vi "main_interface-while-2635_8.3_ZS.vi"() -> ()   [LabVIEW 2014]
uses:
  Instance           1 34Saved   main_interface-while-2635. .vi
  Instance           2 34Saved   main_interface-while-2635. .vi
  Instance           3 34Saved   main_interface-while-2635. .vi
panel:
  out "Vmax":dbl
  out "Jmax":dbl
  in  "Collate Files":bool
  in  "Finger Number":dbl=1.0 min=1.0 max=5.0 step=1.0
  in  "Solar Cell Number":dbl=1.0 min=1.0 max=12.0 step=1.0 format="%0#2_2g"
  in  "Dark Current?":bool
  out "size(s)":i32
  in  "Speed":dbl=1.0
  in  "Serial Configuration":T1={"Baud Rate"=115200, "Parity"=0, "Data Bits"=8, "Stop Bits"=10, "Flow Control"=0} {"Flow Control" items=["None", "XON/XOFF", "RTS/CTS", "XON/XOFF & RTS/CTS", "DTR/DSR", "XON/XOFF & DTR/DSR"]; "Stop Bits" items=["1.0"=10, "1.5"=15, "2.0"=20]; "Data Bits" items=["7"=7, "8"=8]; "Parity" items=["None", "Odd", "Even", "Mark", "Space"]; "Baud Rate" items=["300"=300, "600"=600, "1200"=1200, "2400"=2400, "4800"=4800, "9600"=9600, "19200"=19200]}
  in  "Tab Control":enum32{"Linear Scale", "Log scale"}(tab)
  out "XY Graph":cluster{dbl[], dbl[]}(graph)
  out "XY Graph 2":cluster{dbl[], dbl[]}(graph)
  in  "Start Measurement?":bool
  out "Read Data!":string
  in  "Read File?":bool
  out "S_J_Output (mA/cm^2)":string
  out "J":dbl[](array[numeric])
  out "current_density":dbl[](array[numeric])
  in  "The compliance current (A)":dbl=0.5
  out "stop":bool
  in  "Cancel Measurement?":bool
  out "voltage":dbl[](array[numeric])
  out "current":dbl[](array[numeric])
  out "|voltage|":dbl[](array[numeric])
  out "power":dbl[](array[numeric])
  out "|current|":dbl[](array[numeric])
  out "Measurement Completed?":bool
  in  "Completed, Exit?":bool
  in  "Save to Text file?":bool
  out "path":path
  out "finish":bool
  out "Pmax":dbl
  out "FF":dbl
  out "Isc":dbl
  out "Voc":dbl
  in  "Device Area (cm^2)":dbl=0.06 caption="Step Size (V)" format="%#_6f"
  out "Jsc":dbl
  out "PCE":dbl
  in  "Light  Intensity (mW/cm^2)":dbl=100.0 caption="Step Size (V)" min=2.0
  out "Nth. of Step":i32
  out "error out":errorcluster
  out "S_V_Output (V)":string
  out "S_I_Output (A)":string
  in  "VISA resource name":refnum<visa-resource-name>="COM1"
  out "Voltage increment":dbl
  in  "Final Voltage":dbl=1.0 caption="Final Voltage (V)"
  in  "Step Number":i32=150 caption="Step Size (V)" min=2
  in  "Initial Voltage":dbl=-0.5 caption="Initial Voltage (V)"
  # "(The result will be \nmore accuracy if the\nstep number is larger),"
  # "(0.01-10,the smallar\nvalue,the faster speed)"
  # "Data has been saved!"
  # "To automatically create an Excel Report. \nClick Collate Files and choose all the text files \nwhoose data you want to include in the report"
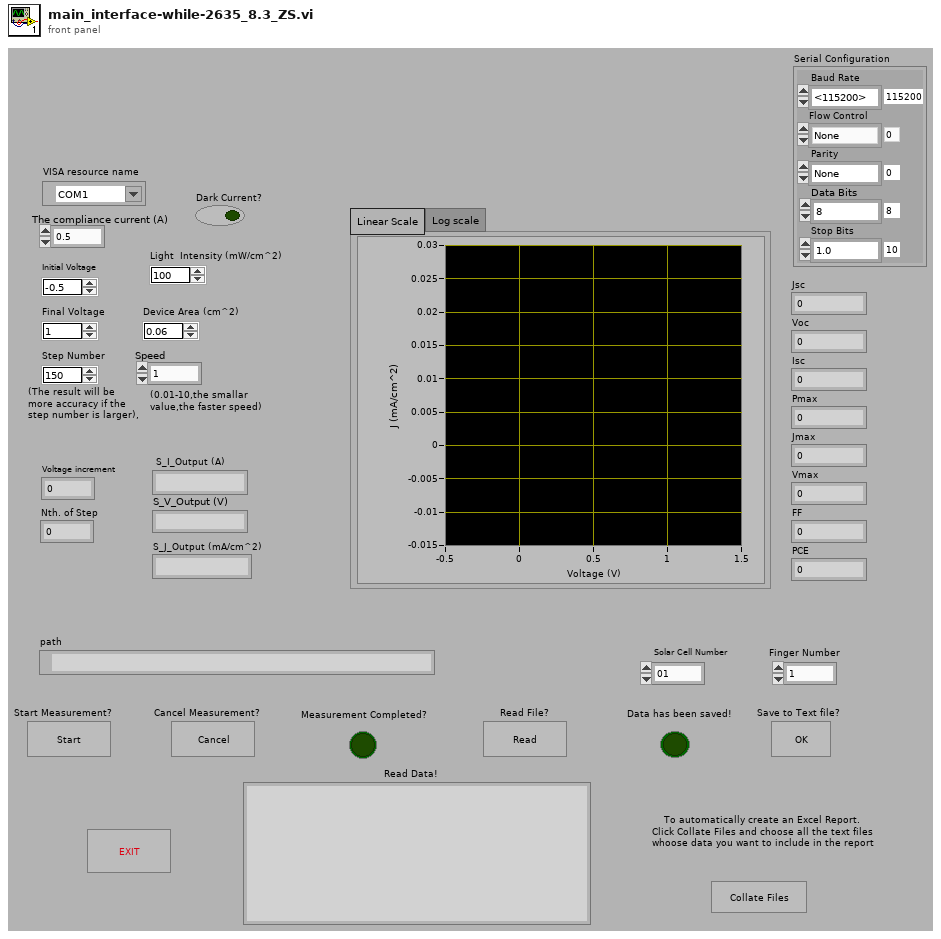
[diagram p1: front panel]
types:
  T1 = cluster{"Baud Rate":u32, "Parity":u16, "Data Bits":u16, "Stop Bits":u16, "Flow Control":u16}
  T2 = enum16{"open", "replace", "create", "open or create", "replace or create", "replace or create with confirmation"}
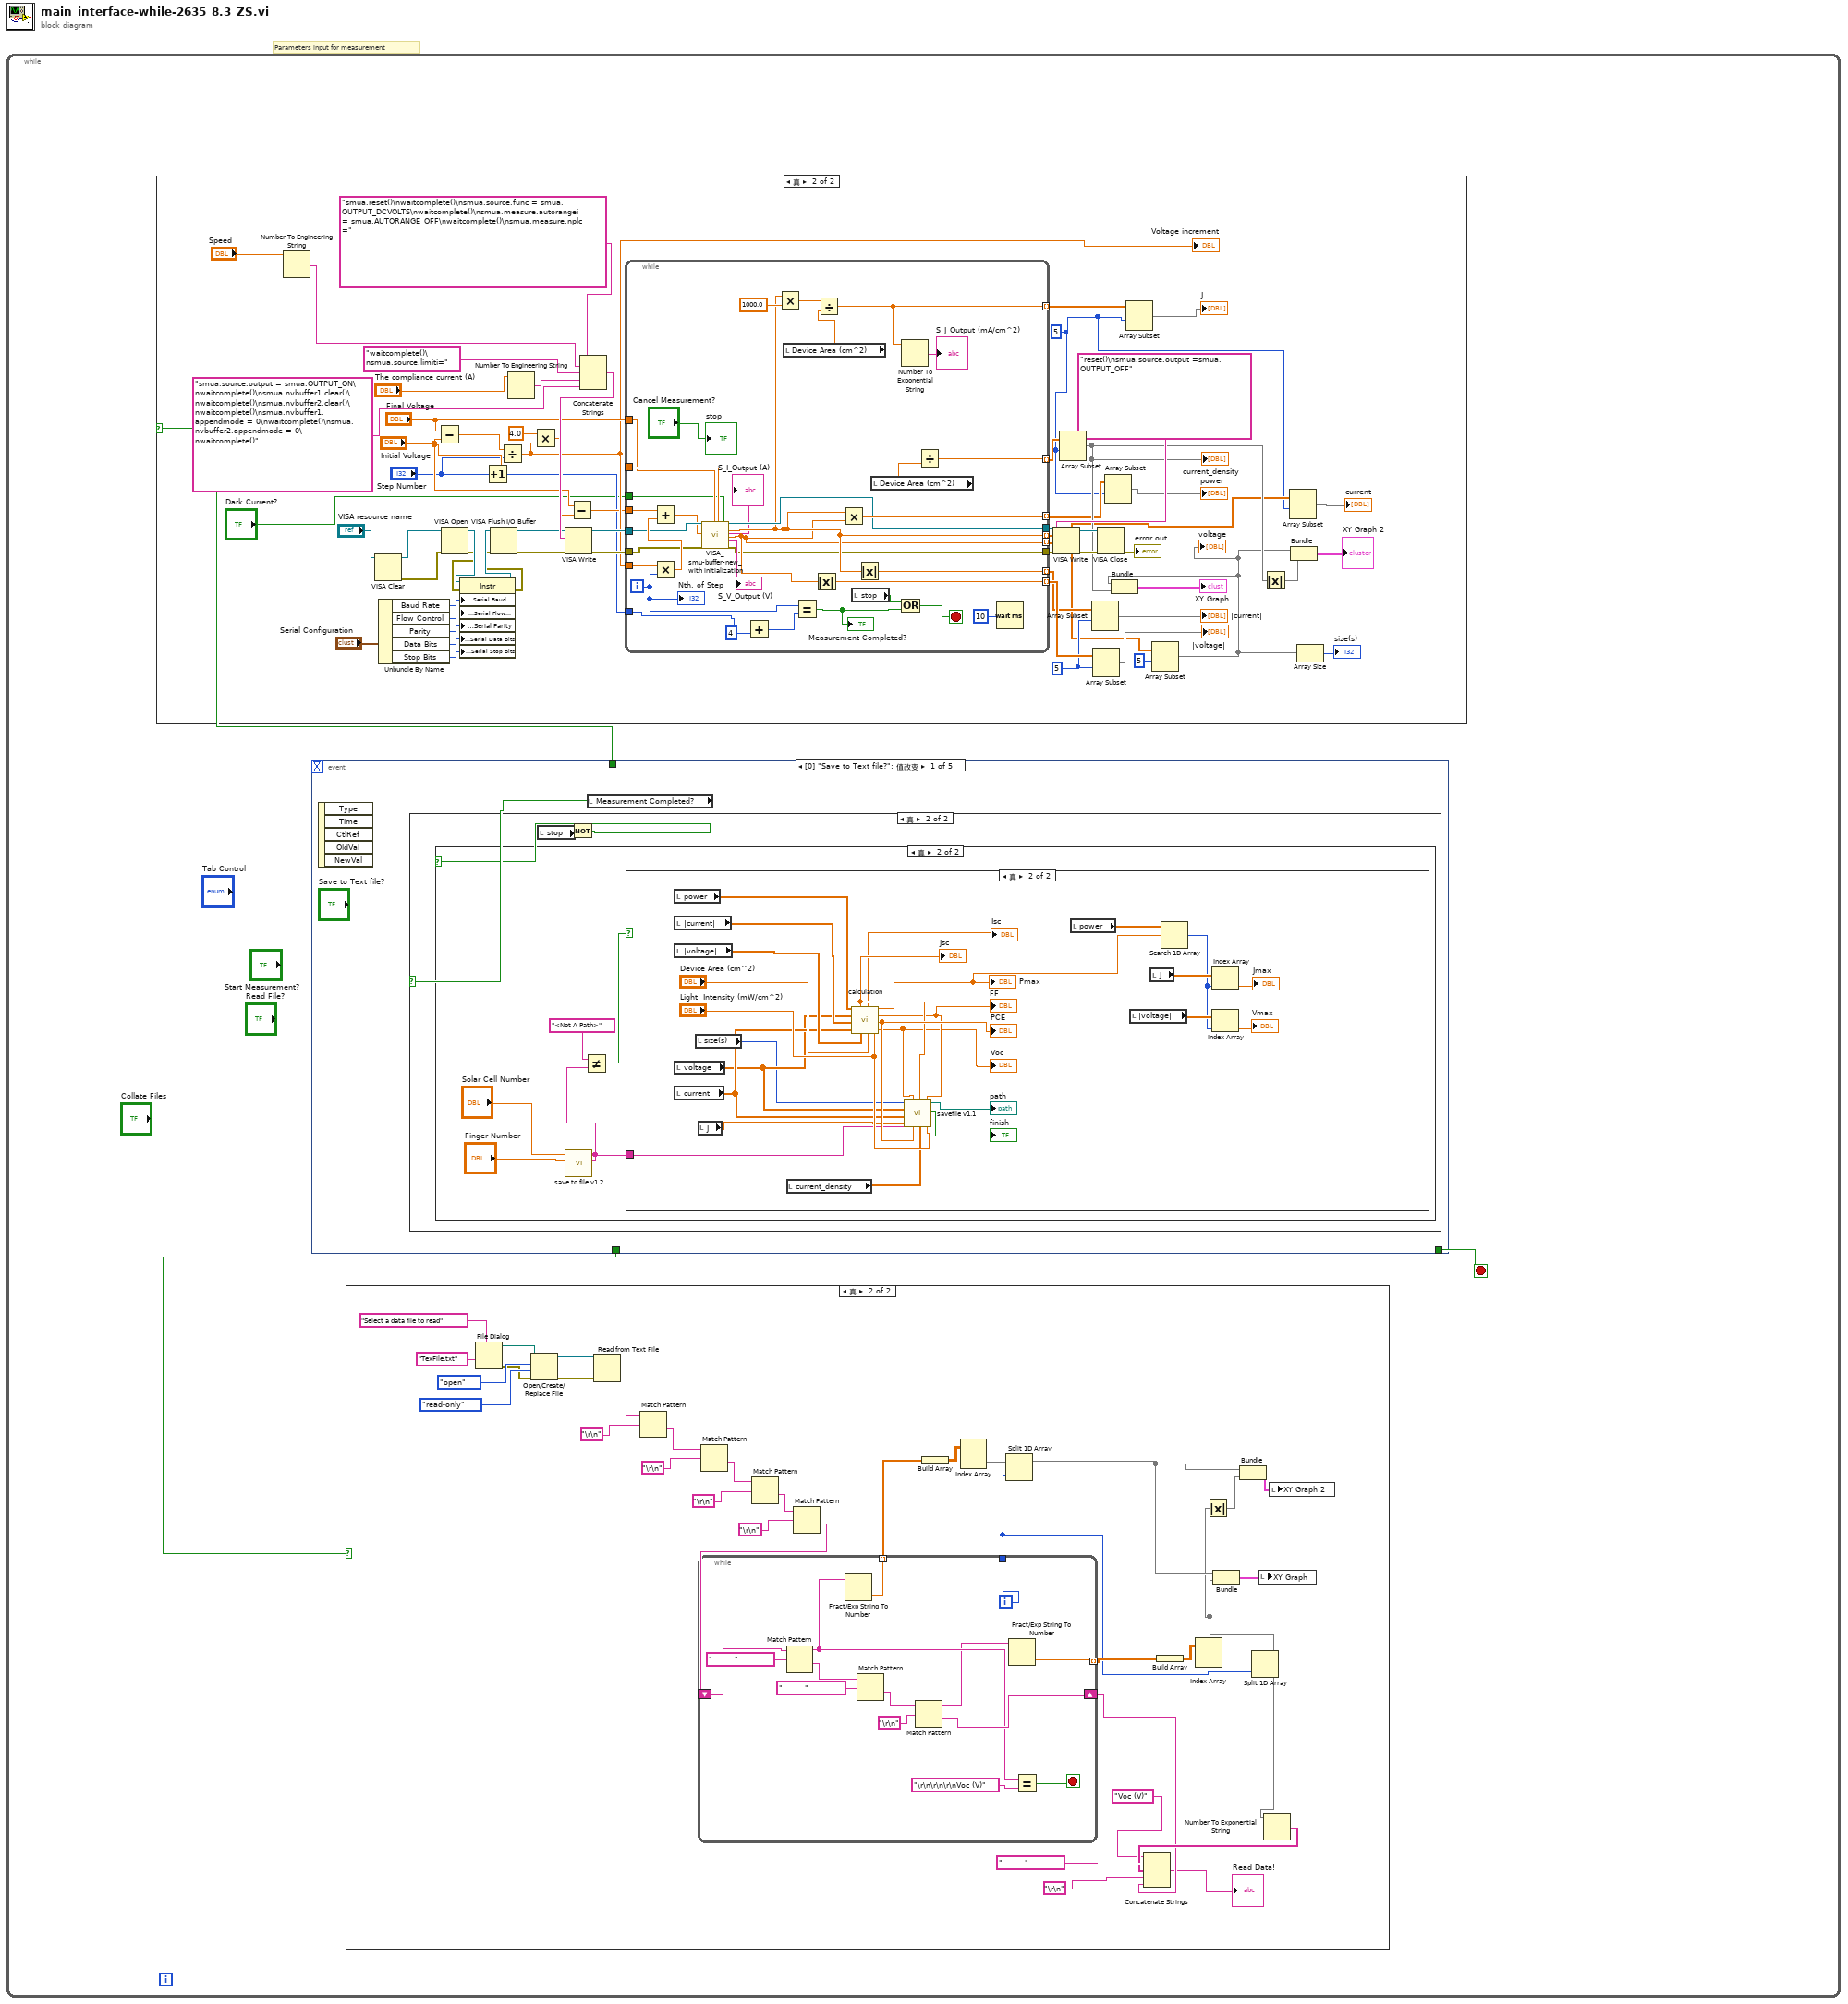
[diagram p0: block diagram]
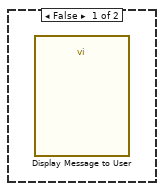
[diagram p4: hidden frame]
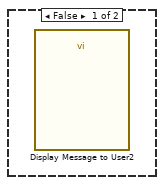
[diagram p5: hidden frame]
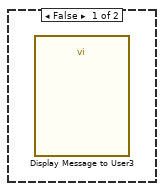
[diagram p6: hidden frame]
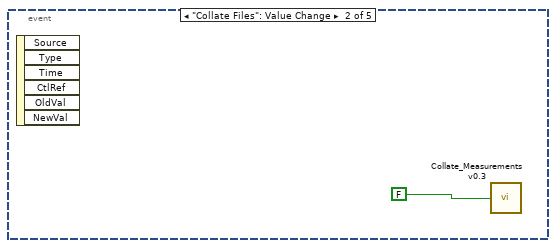
[diagram p7: hidden frame]
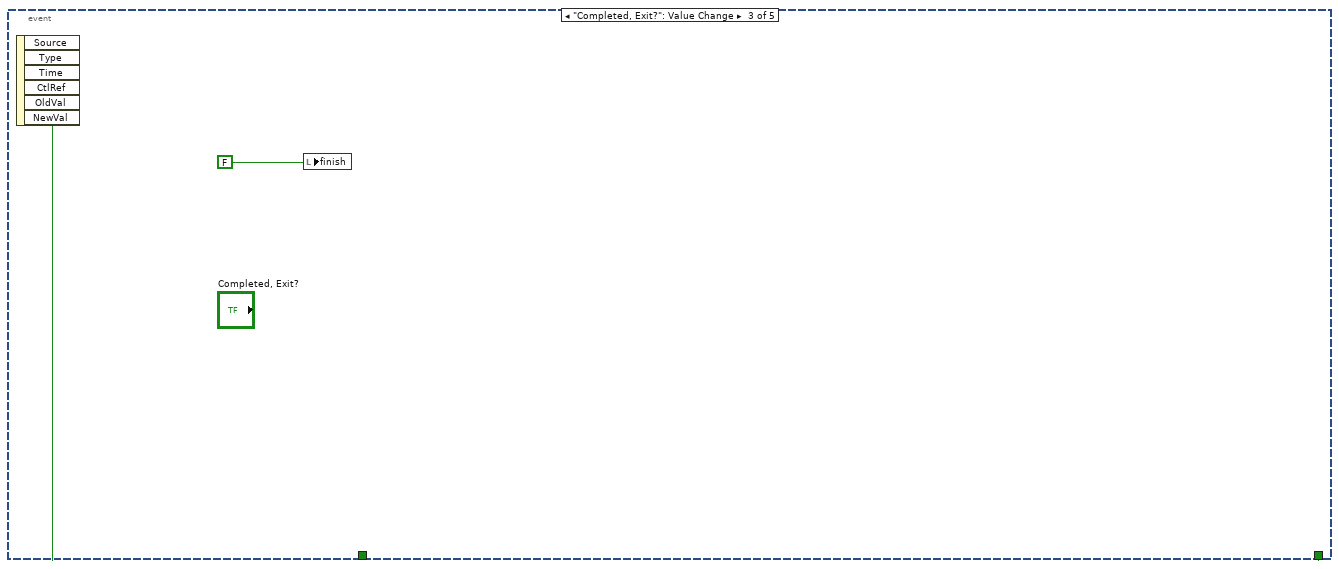
[diagram p8: hidden frame]
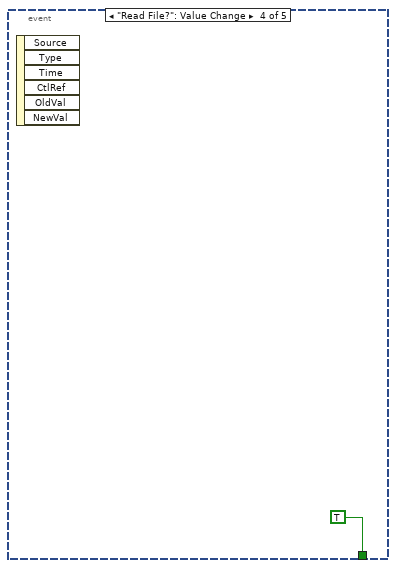
[diagram p9: hidden frame]
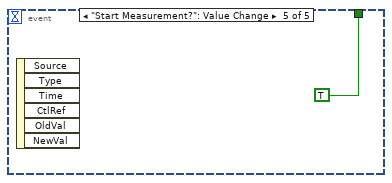
[diagram p10: hidden frame]
diagram:
  # "Parameters input for measurement"
  n1 = while {
    stop <- w3 stop-if-true
    n2 = event shown="[0] \"Save to Text file?\": 值改变" {
      selector: _ -> [_ _ _ _ _]
      dyn-events: _ -> [_ _ _ _ _]
      timeout: _ -> [_ _ _ _ _]
      tunnel: [_ _ w185 _ _] -> w3
      tunnel: [_ _ _ TRUE _] -> w2
      tunnel: [_ _ _ _ TRUE] -> w1
      event "Save to Text file?": Value Change {
        n3 = event-data() -> ()  [unwired: 6 out]
        n4 = local read "Measurement Completed?"() -> (w150:bool)
        n5 = case shown="真" w150 {
          frame False {
            n6 = call "Display Message to User"() -> ()  [unwired: 3 in, 9 out]
          }
          frame True {
            n7 = local read "stop"() -> (w152:bool)
            n8 = Not(x=w152) -> (.not. x?=w151:bool)
            n9 = case shown="真" w151 {
              frame False {
                n10 = call "Display Message to User2"() -> ()  [unwired: 3 in, 9 out]
              }
              frame True {
                n11 = call "save to file v1.2.vi"("Trial Number"="Finger Number", "Solar Cell Number"="Solar Cell Number") -> ("Path"=w155:string)  [unwired: 9 out]
                n12 = Not Equal?(x="<Not A Path>", y=w155) -> (x != y?=w156:bool)
                n13 = case shown="真" w156 {
                  tunnel: w155 -> [_ w169]
                  frame False {
                    n14 = call "Display Message to User3"() -> ()  [unwired: 3 in, 9 out]
                  }
                  frame True {
                    n15 = local read "power"() -> (w173:dbl[])
                    n16 = local read "|current|"() -> (w175:dbl[])
                    n17 = local read "|voltage|"() -> (w177:dbl[])
                    n18 = local read "voltage"() -> (w174:dbl[])
                    n19 = local read "current"() -> (w176:dbl[])
                    n20 = local read "size(s)"() -> (w170:i32)
                    n21 = local read "J"() -> (w165:dbl[])
                    n22 = local read "current_density"() -> (w168:dbl[])
                    n23 = call "calculation.vi"("power"=w173, "voltage"=w174, "|current|"=w175, "current"=w176, "|voltage|"=w177, "Device Area (cm^2)"="Device Area (cm^2)", "Light  Intensity (mW/cm^2)"="Light  Intensity (mW/cm^2)") -> ("Jsc"=w180:dbl, "Isc"=→"Isc":dbl, "IVmax"=w163:dbl, "FF"=w178:dbl, "Pce"=w181:dbl, "Voc"=w166:dbl)  [unwired: 15 out]
                    "Pmax" <- w163
                    "FF" <- w178
                    "Voc" <- w166
                    "Jsc" <- w180
                    "PCE" <- w181
                    n24 = call "savefile v1.1.vi"("Length of array"=w170, "voltage"=w174, "current"=w176, "J"=w165, "path of file"=w169, "Voc"=w166, "Power convertion efficiency"=w181, "Jsc"=w180, "current density"=w168, "FF"=w178, "Lamp Power"="Light  Intensity (mW/cm^2)") -> ("path"=→"path":path, "x = y?"=→"finish":bool)  [unwired: 15 out]
                    n25 = local read "power"() -> (w164:dbl[])
                    n26 = local read "|voltage|"() -> (w161:dbl[])
                    n27 = local read "J"() -> (w162:dbl[])
                    n28 = Search 1D Array(1D array=w164, element=w163) -> (index of element=w160:i32)  [unwired: 1 out]
                    n29 = Index Array(array=w162, index=w160) -> (element=→"Jmax":dbl)
                    n30 = Index Array(array=w161, index=w160) -> (element=→"Vmax":dbl)
                  }
                }
              }
            }
          }
        }
      }
      event "Collate Files": Value Change {
        n31 = event-data() -> ()  [unwired: 7 out]
        n32 = call "Collate_Measurements v0.3.vi"("Collate Files"=FALSE) -> ()  [unwired: 1 out]
      }
      event "Completed, Exit?": Value Change {
        n33 = event-data() -> ("NewVal"=w185:bool)  [unwired: 6 out]
        n34 = local write "finish"(FALSE) -> ()
      }
      event "Read File?": Value Change {
        n35 = event-data() -> ()  [unwired: 7 out]
      }
      event "Start Measurement?": Value Change {
        n36 = event-data() -> ()  [unwired: 7 out]
      }
    }
    n37 = case shown="真" w1 {
      frame False {
      }
      frame True {
        w26 = 5 ("index")
        w21 = 5 ("index")
        n38 = Number To Engineering String(4:"Speed") -> (0:w15:string)  [unwired: 3 out]
        n39 = VISA Clear(VISA resource name="VISA resource name") -> (VISA resource name out=w38:refnum<visa-resource-name>, error out=w40:errorcluster)  [unwired: 1 in]
        n40 = Unbundle By Name("Serial Configuration") -> ("Baud Rate"=w45:u32, "Flow Control"=w44:u16, "Parity"=w43:u16, "Data Bits"=w42:u16, "Stop Bits"=w41:u16)
        n41 = Subtract(x="Final Voltage", y="Initial Voltage") -> (x-y=w13:dbl)
        n42 = VISA Open(error in (no error)=w40, VISA resource name=w38) -> (VISA resource name=w49:refnum<visa-resource-name>, error out=w47:errorcluster)  [unwired: 3 out]
        n43 = property class="Instr"(reference=w49, error in=w47, "Serial Settings:Serial Baud Rate"=w45, "Serial Settings:Serial Flow Control"=w44, "Serial Settings:Serial Parity"=w43, "Serial Settings:Serial Data Bits"=w42, "Serial Settings:Serial Stop Bits"=w41) -> (reference out=w48:refnum<visa-resource-name>, error out=w46:errorcluster)
        n44 = Increment(x="Step Number") -> (x+1=w5:i32)
        n45 = VISA Flush I/O Buffer(VISA resource name=w48, error in (no error)=w46) -> (VISA resource name out=w55:refnum<visa-resource-name>, error out=w56:errorcluster)  [unwired: 1 out]
        n46 = Divide(x=w13, y="Step Number") -> (x/y=w11:dbl)
        "Voltage increment" <- w11
        n47 = Number To Engineering String(4:"The compliance current (A)") -> (0:w17:string)  [unwired: 3 out]
        n48 = Multiply(x=4.0, y=w11) -> (x*y=w7:dbl)
        n49 = Subtract(x="Initial Voltage", y=w7) -> (x-y=w9:dbl)
        n50 = Concatenate Strings("smua.reset()\nwaitcomplete()\nsmua.source.func = smua.OUTPUT_DCVOLTS\nwaitcomplete()\nsmua.measure.autorangei = smua.AUTORANGE_OFF\nwaitcomplete()\nsmua.measure.nplc =", w15, "waitcomplete()\nsmua.source.limiti=", w17, "smua.source.output = smua.OUTPUT_ON\nwaitcomplete()\nsmua.nvbuffer1.clear()\nwaitcomplete()\nsmua.nvbuffer2.clear()\nwaitcomplete()\nsmua.nvbuffer1.appendmode = 0\nwaitcomplete()\nsmua.nvbuffer2.appendmode = 0\nwaitcomplete()" ("string")) -> (w60:string)
        n51 = VISA Write(VISA resource name=w55, write buffer=w60, error in (no error)=w56) -> (VISA resource name out=w57:refnum<visa-resource-name>, error out=w58:errorcluster)  [unwired: 1 out]
        n52 = while {
          tunnel: w57 -> [w82]
          tunnel: w58 -> [w80]
          tunnel: [w74] -> w65
          tunnel: [w79] -> w64
          tunnel: w11 -> [w99]
          tunnel: w9 -> [w98]
          tunnel: [w78] -> w22 mode=indexing
          tunnel: [w76] -> w25 mode=indexing
          tunnel: [w96] -> w32 mode=indexing
          tunnel: [w90] -> w28 mode=indexing
          tunnel: [w95] -> w30 mode=indexing
          tunnel: w5 -> [w69]
          tunnel: [w88] -> w34 mode=indexing
          tunnel: [w84] -> w36 mode=indexing
          tunnel: "Initial Voltage" -> [w71]
          tunnel: "Final Voltage" -> [w70]
          tunnel: "Dark Current?" -> [w66]
          i -> [w72]
          stop <- w94 stop-if-true
          n53 = Multiply(x=w99, y=w72) -> (x*y=w97:dbl)
          n54 = Add(x=w98, y=w97) -> (x+y=w81:dbl)
          n55 = call "VISA_smu-buffer-new_with initialization.vi"("VISA resource name in"=w82, "Voltage Source Level (V)"=w81, "error in (no error)"=w80, "End voltage"=w70, "Initial voltage"=w71, "Dark Current"=w66) -> ("VISA resource name out"=w79:refnum<visa-resource-name>, "F_I_Output (A)"=w78:dbl, "S_I_Output (A)"=→"S_I_Output (A)":string, "F_V_Output (V)"=w76:dbl, "S_V_Output (V)"=→"S_V_Output (V)":string, "error out"=w74:errorcluster)  [unwired: 16 out]
          n56 = Add(x=w69, y=4) -> (x+y=w67:i32)
          n57 = Multiply(x=w78, y=1000.0) -> (x*y=w86:dbl)
          n58 = local read "Device Area (cm^2)"() -> (w85:dbl)
          n59 = Equal?(x=w72, y=w67) -> (x = y?=w91:bool)
          "Measurement Completed?" <- w91
          n60 = Absolute Value(x=w76) -> (abs(x)=w95:dbl)
          n61 = Divide(x=w86, y=w85) -> (x/y=w84:dbl)
          n62 = Multiply(x=w78, y=w76) -> (x*y=w96:dbl)
          n63 = local read "stop"() -> (w92:bool)
          n64 = Absolute Value(x=w78) -> (abs(x)=w90:dbl)
          n65 = local read "Device Area (cm^2)"() -> (w89:dbl)
          n66 = Or(x=w92, y=w91) -> (x .or. y?=w94:bool)
          n67 = Number To Exponential String(number=w84) -> (E-format string=→"S_J_Output (mA/cm^2)":string)  [unwired: 3 out]
          n68 = Divide(x=w78, y=w89) -> (x/y=w88:dbl)
          n69 = Wait (ms)(milliseconds to wait=u32 10) -> ()  [unwired: 1 out]
          "Nth. of Step" <- w72
          "stop" <- "Cancel Measurement?"
        }
        n70 = VISA Write(VISA resource name=w64, write buffer="reset()\nsmua.source.output =smua.OUTPUT_OFF", error in (no error)=w65) -> (VISA resource name out=w62:refnum<visa-resource-name>, error out=w63:errorcluster)  [unwired: 1 out]
        n71 = Array Subset(array=w34, index=w21) -> (w33:dbl[])  [unwired: 1 in]
        "current_density" <- w33
        n72 = Array Subset(array=w28, index=w26) -> (→"|current|":dbl[])  [unwired: 1 in]
        n73 = Array Subset(array=w30, index=w26) -> (→"|voltage|":dbl[])  [unwired: 1 in]
        n74 = VISA Close(VISA resource name=w62, error in (no error)=w63) -> (error out=→"error out":errorcluster)
        n75 = Array Subset(array=w32, index=w21) -> (→"power":dbl[])  [unwired: 1 in]
        n76 = Array Subset(array=w36, index=w21) -> (→"J":dbl[])  [unwired: 1 in]
        n77 = Array Subset(array=w25, index=5) -> (w19:dbl[])  [unwired: 1 in]
        "voltage" <- w19
        n78 = Bundle "Bundle"(w19, w33) -> (→"XY Graph":cluster{dbl[], dbl[]})  [unwired: 1 out]
        n79 = Absolute Value(x=w33) -> (abs(x)=w51:dbl[])
        n80 = Array Subset(array=w22, index=w21) -> (→"current":dbl[])  [unwired: 1 in]
        n81 = Bundle "Bundle"(w19, w51) -> (→"XY Graph 2":cluster{dbl[], dbl[]})  [unwired: 1 out]
        n82 = Array Size(array=w19) -> (size(s)=→"size(s)":i32)
      }
    }
    n83 = case shown="真" w2 {
      frame False {
      }
      frame True {
        n84 = File Dialog(7:"Select a data file to read" ("prompt"), 9:"TexFile.txt" ("default name")) -> (0:w129:errorcluster, 3:w133:path)  [unwired: 1 in, 6 out]
        n85 = Open/Create/Replace File(file path (use dialog)=w133, error in=w129, operation (0:open)=T2."open", access (0:read/write)=enum16{"read/write", "read-only", "write-only"}."read-only") -> (refnum out=w130:refnum<file>, error out=w128:errorcluster)  [unwired: 3 out]
        n86 = Read from Text File(file (use dialog)=w130, error in=w128) -> (text=w127:string)  [unwired: 5 out]
        n87 = Match Pattern(string=w127, regular expression="\r\n") -> (after substring=w123:string)  [unwired: 4 out]
        n88 = Match Pattern(string=w123, regular expression="\r\n") -> (after substring=w122:string)  [unwired: 4 out]
        n89 = Match Pattern(string=w122, regular expression="\r\n") -> (after substring=w120:string)  [unwired: 4 out]
        n90 = Match Pattern(string=w120, regular expression="\r\n") -> (after substring=w119:string)  [unwired: 4 out]
        n91 = while {
          shift-right: [w143] -> w109
          shift-left: w119 -> [w144]
          tunnel: [w140] -> w116 mode=indexing
          tunnel: [w138] -> w113 mode=indexing
          tunnel: [w136] -> w101
          i -> [w136]
          stop <- w142 stop-if-true
          n92 = Match Pattern(string=w144, regular expression="        ") -> (before substring=w141:string, after substring=w149:string)  [unwired: 3 out]
          n93 = Fract/Exp String To Number(string=w141) -> (number=w140:dbl)  [unwired: 4 out]
          n94 = Match Pattern(string=w149, regular expression="        ") -> (after substring=w148:string)  [unwired: 4 out]
          n95 = Match Pattern(string=w148, regular expression="\r\n") -> (before substring=w139:string, after substring=w143:string)  [unwired: 3 out]
          n96 = Fract/Exp String To Number(string=w139) -> (number=w138:dbl)  [unwired: 4 out]
          n97 = Equal?(x=w141, y="\r\n\r\n\r\nVoc (V)") -> (x = y?=w142:bool)
        }
        n98 = Build Array(w116) -> (w118:dbl[][])
        n99 = Index Array(array=w118) -> (element=w117:dbl[])  [unwired: 2 in]
        n100 = Split 1D Array(array=w117, index=w101) -> (first subarray=w105:dbl[])  [unwired: 1 out]
        n101 = Build Array(w113) -> (w115:dbl[][])
        n102 = Index Array(array=w115) -> (element=w114:dbl[])  [unwired: 2 in]
        n103 = Split 1D Array(array=w114, index=w101) -> (first subarray=w103:dbl[], second subarray=w111:dbl[])
        n104 = Absolute Value(x=w103) -> (abs(x)=w104:dbl[])
        n105 = Bundle(w105, w103) -> (w106:cluster{dbl[], dbl[]})  [unwired: 1 out]
        n106 = Bundle(w105, w104) -> (w102:cluster{dbl[], dbl[]})  [unwired: 1 out]
        n107 = local write "XY Graph"(w106) -> ()
        n108 = Number To Exponential String(number=w111) -> (E-format string=w110:string[])  [unwired: 3 out]
        n109 = Concatenate Strings("Voc (V)" ("y"), "        " ("string"), w110, "\r\n", w109) -> (→"Read Data!":string)
        n110 = local write "XY Graph 2"(w102) -> ()
      }
    }
  }
